vi "Acquisizione corse.vi"() -> ()   [LabVIEW 2017]
uses:
  <vilib>/DAQmx/read.llb/DAQmx Read (Analog 1D Wfm NChan NSamp).vi
  <vilib>/DAQmx/configure/timing.llb/DAQmx Timing (Sample Clock).vi
  <vilib>/DAQmx/miscellaneous.llb/DAQmx Fill In Error Info.vi
  <vilib>/Waveform/WDTOps.llb/WDT Index Channel DBL.vi
  <vilib>/Waveform/WDTOps.llb/WDT Append Waveforms DBL.vi
  <vilib>/measure/maspectr.llb/FFT Spectrum (Mag-Phase) for 1 Chan.vi
  <vilib>/measure/maspectr.llb/FFT Power Spectrum and PSD for 1 Chan.vi
  <vilib>/measure/NI_MAPro.lvlib
panel:
  out "salvataggio":bool
  out "fotocellula 2":bool
  out "fotocellula 1":bool
  in  "?":bool
  in  "directory":path
  in  "Massa":string="_"
  in  "Source start":i32=2
  in  "Soglia Start":dbl=4.0
  in  "Source Stop":i32=2
  in  "Soglia Stop":dbl=4.0
  in  "error in (no error)":errorcluster
  out "error out":errorcluster
  in  "Save":bool
  in  "samples per channel":i32=1000
  in  "sample mode":i32(ring)=10178 items=["Finite Samples"=10178, "Continuous Samples"=10123, "Hardware Timed Single Point"=12522]
  in  "rate":dbl=1000.0 format="%0.2f"
  in  "canale di acquisizione":refnum<k21>="NastroTrasportatore"
  in  "Lower Cut-Off":dbl=100.0
  in  "Tab Control":enum32{"signals", "PSD", "FFT"}(tab)
  out "Load_Cell":waveform(dbl)(graph)
  out "Photocell A":waveform(dbl)(graph)
  out "Photocell B":waveform(dbl)(graph)
  out "Load_Cell filtered":dynamicdata(graph)
  out "PSD":cluster{"f0":dbl, "df":dbl, "magnitude":dbl[]}(graph)
  out "Magnitude":cluster{"f0":dbl, "df":dbl, "magnitude":dbl[]}(graph)
  out "Phase":cluster{"f0":dbl, "df":dbl, "phase":dbl[]}(graph)
  # "45 m/min\n80 m/min"
  # "0,42 m corsa totale"
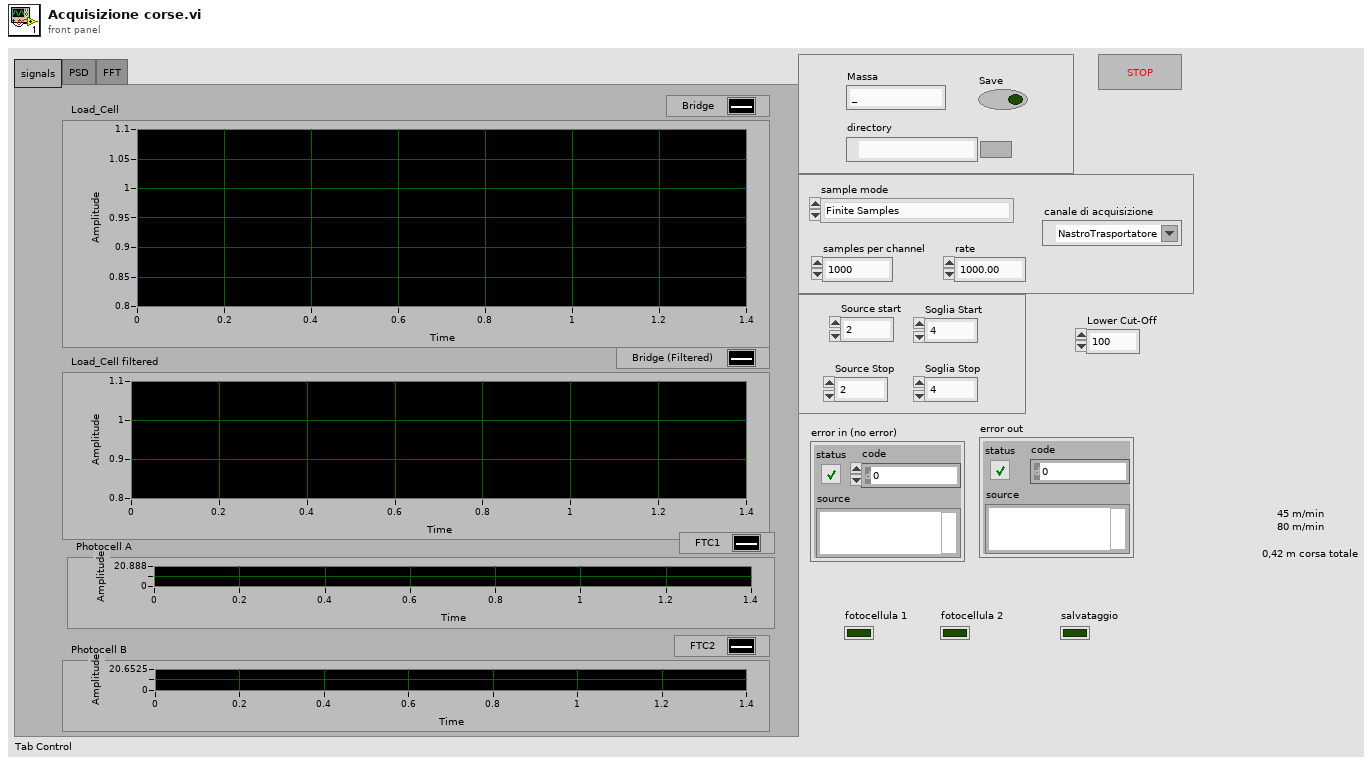
[diagram p1: front panel]
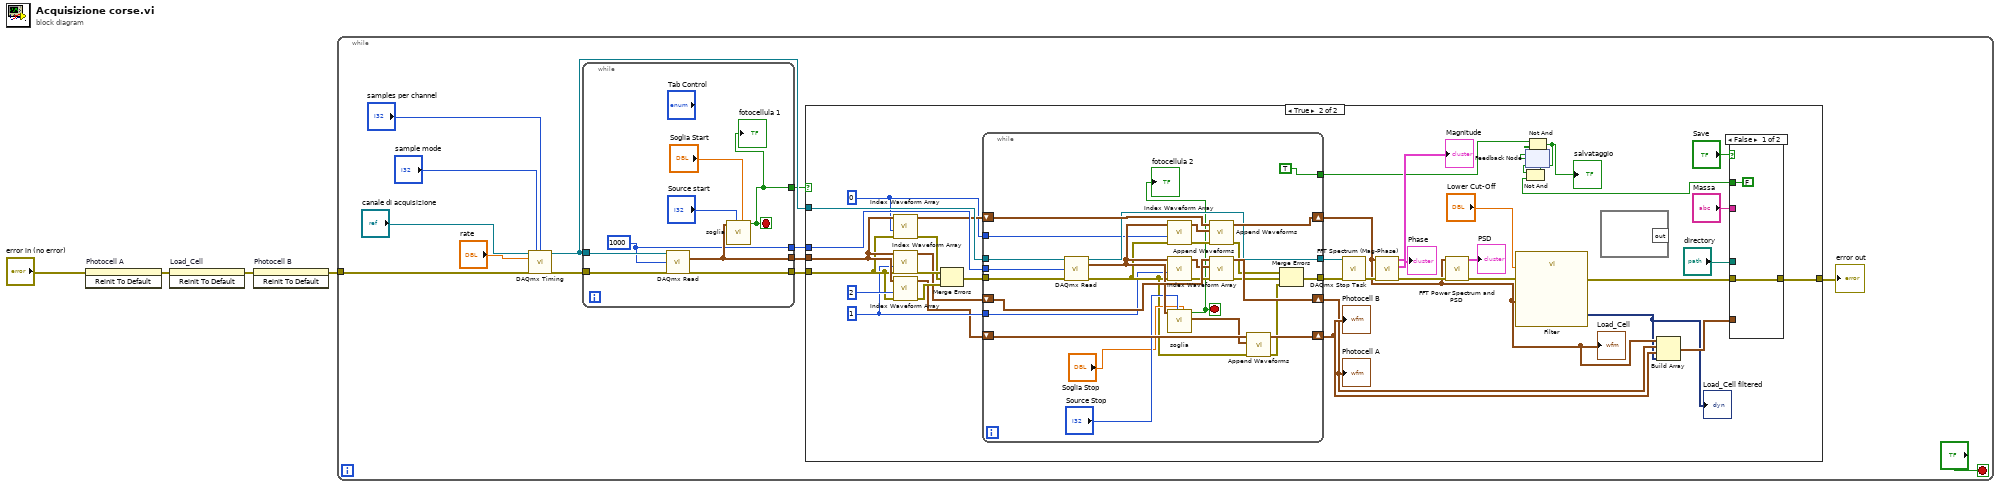
[diagram p0: block diagram]
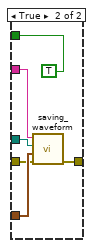
[diagram p3: hidden frame]
diagram:
  n1 = invoke on="Photocell A" class="WFGraph (strict)" method="Reinit To Default"(error in="error in (no error)") -> (error out=w3:errorcluster)  [unwired: 2 in, 2 out]
  n2 = invoke on="Load_Cell" class="WFGraph (strict)" method="Reinit To Default"(error in=w3) -> (error out=w2:errorcluster)  [unwired: 2 in, 2 out]
  n3 = invoke on="Photocell B" class="WFGraph (strict)" method="Reinit To Default"(error in=w2) -> (error out=w1:errorcluster)  [unwired: 2 in, 2 out]
  n4 = while {
    tunnel: w1 -> [w6]
    stop <- "?" stop-if-true
    n5 = call-poly <vilib>:"DAQmx Timing.vi"("task/channels in"="canale di acquisizione", "sample mode"="sample mode", "samples per channel"="samples per channel", "rate"="rate", "error in"=w6) -> ("task out"=w12:refnum<k21>, "error out"=w11:errorcluster)  [unwired: 9 in]
    n6 = while {
      tunnel: [w18] -> w5
      tunnel: [w25] -> w16
      tunnel: w12 -> [w24]
      tunnel: [w23] -> w15
      tunnel: w11 -> [w20]
      tunnel: [w19] -> w14
      stop <- w18 stop-if-true
      w23 = 1000 ("number of samples per channel")
      n7 = call-poly <vilib>:"DAQmx Read.vi"("task/channels in"=w24, "number of samples per channel"=w23, "error in"=w20) -> ("data"=w25:waveform(dbl)[], "error out"=w19:errorcluster)  [unwired: 10 in, 1 out]
      n8 = call "soglia.vi"("valore di controllo"="Soglia Start", "index"="Source start", "waveform_in"=w25) -> ("Boolean"=w18:bool)  [unwired: 7 in, 1 out]
      "fotocellula 1" <- w18
    }
    n9 = case shown="True" w5 {
      tunnel: w16 -> [_ w63]
      tunnel: w12 -> [_ w62]
      tunnel: w15 -> [_ w61]
      tunnel: w14 -> [w26 w57]
      tunnel: [w26 w52] -> w13
      frame False {
      }
      frame True {
        w45 = 1 ("index")
        w46 = 0 ("index")
        n10 = call-poly <vilib>:"Index Waveform Array.vi"("error in (no error)"=w57, "index"=w46, "waveform array"=w63) -> ("error out"=w55:errorcluster, "waveform"=w50:waveform(dbl))  [unwired: 7 in]
        n11 = call-poly <vilib>:"Index Waveform Array.vi"("error in (no error)"=w57, "index"=w45, "waveform array"=w63) -> ("error out"=w56:errorcluster, "waveform"=w51:waveform(dbl))  [unwired: 7 in]
        n12 = call-poly <vilib>:"Index Waveform Array.vi"("error in (no error)"=w57, "index"=2, "waveform array"=w63) -> ("error out"=w54:errorcluster, "waveform"=w43:waveform(dbl))  [unwired: 7 in]
        n13 = Merge Errors(w56, w55, w54) -> (w53:errorcluster)
        n14 = while {
          shift-right: [w97] -> w28
          shift-left: w50 -> [w98]
          shift-right: [w94] -> w42
          shift-left: w51 -> [w96]
          shift-right: [w92] -> w58
          shift-left: w43 -> [w93]
          tunnel: w62 -> [w91]
          tunnel: w61 -> [w90]
          tunnel: [w89] -> w60
          tunnel: w53 -> [w84]
          tunnel: [w77] -> w44
          tunnel: w46 -> [w76]
          tunnel: w45 -> [w75]
          tunnel: [TRUE] -> w33
          stop <- w74 stop-if-true
          n15 = call-poly <vilib>:"DAQmx Read.vi"("task/channels in"=w91, "number of samples per channel"=w90, "error in"=w84) -> ("task out"=w89:refnum<k21>, "data"=w88:waveform(dbl)[], "error out"=w81:errorcluster)  [unwired: 10 in]
          n16 = call-poly <vilib>:"Index Waveform Array.vi"("error in (no error)"=w81, "index"=w76, "waveform array"=w88) -> ("error out"=w82:errorcluster, "waveform"=w99:waveform(dbl))  [unwired: 7 in]
          n17 = call-poly <vilib>:"Index Waveform Array.vi"("error in (no error)"=w81, "index"=w75, "waveform array"=w88) -> ("error out"=w83:errorcluster, "waveform"=w95:waveform(dbl))  [unwired: 7 in]
          n18 = call "soglia.vi"("valore di controllo"="Soglia Stop", "index"="Source Stop", "waveform_in"=w88) -> ("waveform_out_single"=w87:waveform(dbl), "Boolean"=w74:bool)  [unwired: 7 in]
          "fotocellula 2" <- w74
          n19 = call-poly <vilib>:"Append Waveforms.vi"("error in (no error)"=w82, "waveform B"=w99, "waveform A"=w98) -> ("error out"=w80:errorcluster, "waveform out"=w97:waveform(dbl))  [unwired: 7 in]
          n20 = call-poly <vilib>:"Append Waveforms.vi"("error in (no error)"=w83, "waveform B"=w95, "waveform A"=w96) -> ("error out"=w79:errorcluster, "waveform out"=w94:waveform(dbl))  [unwired: 7 in]
          n21 = call-poly <vilib>:"Append Waveforms.vi"("error in (no error)"=w81, "waveform B"=w87, "waveform A"=w93) -> ("error out"=w78:errorcluster, "waveform out"=w92:waveform(dbl))  [unwired: 7 in]
          n22 = Merge Errors(w80, w79, w78) -> (w77:errorcluster)
        }
        "Load_Cell" <- w28
        "Photocell A" <- w42
        "Photocell B" <- w58
        n23 = call <vilib>:"DAQmx Stop Task.vi"("task/channels in"=w60, "error in"=w44) -> ("error out"=w37:errorcluster)  [unwired: 12 in, 1 out]
        n24 = call-poly <vilib>:"FFT Spectrum (Mag-Phase).vi"("error in (no error)"=w37, "time signal"=w28) -> ("error out"=w36:errorcluster, "phase"=→"Phase":cluster{"f0":dbl, "df":dbl, "phase":dbl[]}, "magnitude"=→"Magnitude":cluster{"f0":dbl, "df":dbl, "magnitude":dbl[]})  [unwired: 5 in, 2 out]
        n25 = call-poly <vilib>:"FFT Power Spectrum and PSD.vi"("error in (no error)"=w36, "time signal"=w28) -> ("error out"=w35:errorcluster, "Power Spectrum / PSD"=→"PSD":cluster{"f0":dbl, "df":dbl, "magnitude":dbl[]})  [unwired: 6 in, 2 out]
        n26 = call "Filter"("error in (no error)"=w35, "Lower Cut-Off"="Lower Cut-Off", "Signal"=w28) -> ("error out"=w40:errorcluster, "Filtered Signal"=w27:dynamicdata)  [unwired: 7 in]
        "Load_Cell filtered" <- w27
        n27 = feedback #1() -> (w30:bool)  [unwired: 1 in]
        n28 = Not And(1:w30, 2:w33) -> (0:w29:bool)
        "salvataggio" <- w29
        n29 = formula code=""() -> ()  [unwired: 1 out]
        n30 = Build Array(w28, w42, w58, w27) -> (w59:waveform(dbl)[])
        n31 = case shown="False" "Save" {
          tunnel: w59 -> [_ w72]
          tunnel: w40 -> [w66 w71]
          tunnel: [w66 w70] -> w52
          tunnel: "directory" -> [_ w69]
          tunnel: "Massa" -> [_ w68]
          tunnel: [FALSE TRUE] -> w32
          frame False {
          }
          frame True {
            n32 = call "saving_waveform.vi"("error in (no error)"=w71, "Array"=w72, "directory"=w69, "Massa"=w68) -> ("error out"=w70:errorcluster)  [unwired: 7 in]
          }
        }
        n33 = Not And(1:w32, 2:w29) -> (0:w31:bool)
        n34 = feedback-in #1(w31) -> ()
      }
    }
    "error out" <- w13
  }
